vi "Main.vi"() -> ()   [LabVIEW 2017]
uses:
  Variable globale.vi
  ICNC/ICNC2.lvlib
panel:
  out "Speed Z":dbl
  out "Speed X":dbl
  out "Speed Y":dbl
  in  "Load Settings":bool
  in  "x-":bool
  in  "x+":bool
  out "Z Position":i32
  out "X Position":i32
  out "Y Position":i32
  in  "z+":bool
  in  "z-":bool
  in  "y+":bool
  in  "y-":bool
  in  "z+y+":bool
  in  "z-y+":bool
  in  "z-y-":bool
  in  "z+y-":bool
  in  "Speed in mm/s":dbl(slide) scale=0.0..1000.0
  in  "Go1":bool
  in  "Z":dbl
  in  "Y":dbl
  in  "X":dbl
  in  "System settings":bool
  out "Unlocked":bool
  out "Connected":bool
  in  "PARAM DLG":bool
  in  "stop motors":bool
  in  "Pos0":bool
  in  "stop":bool
  # "POSITION"
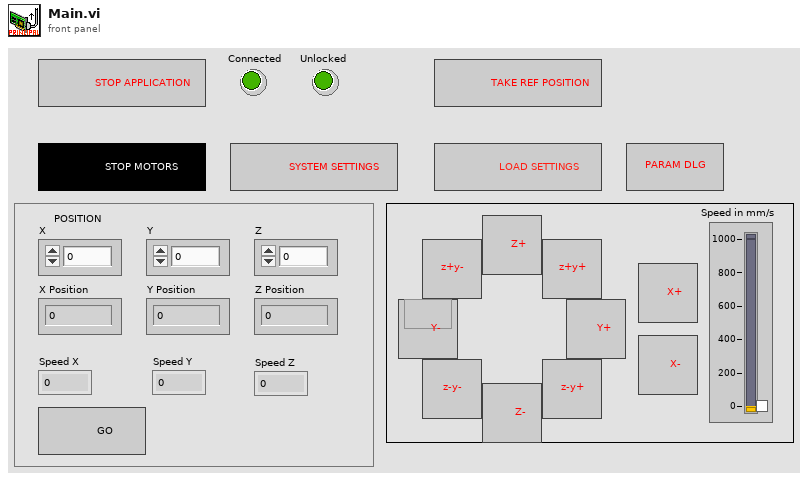
[diagram p1: front panel]
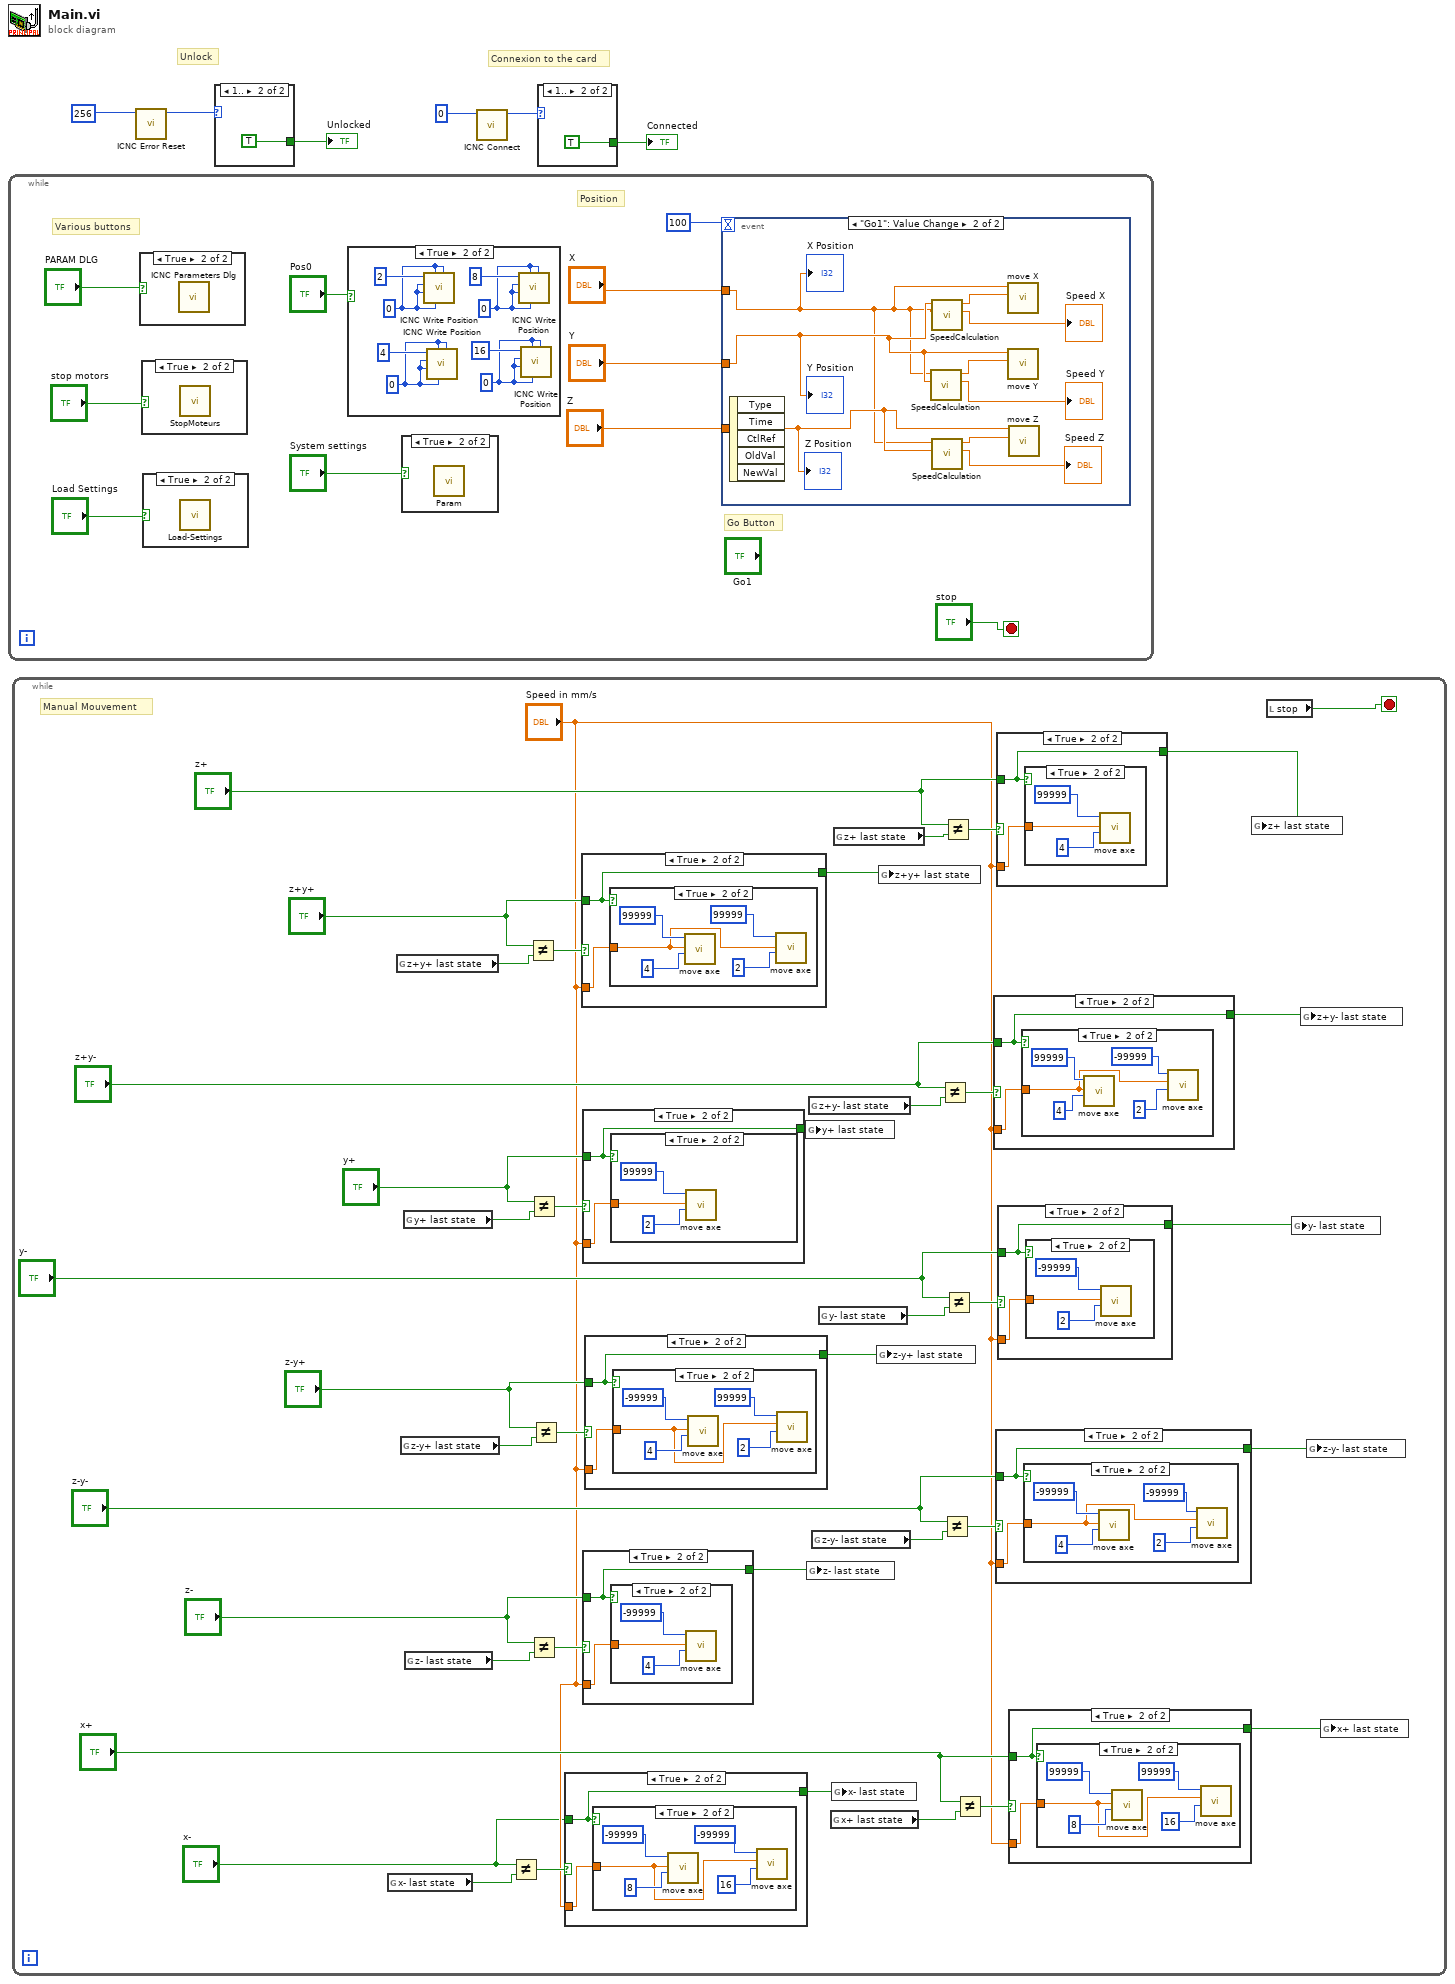
[diagram p0: block diagram]
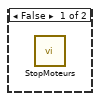
[diagram p3: hidden frame]
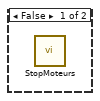
[diagram p5: hidden frame]
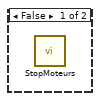
[diagram p7: hidden frame]
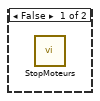
[diagram p9: hidden frame]
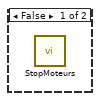
[diagram p11: hidden frame]
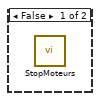
[diagram p13: hidden frame]
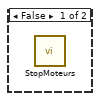
[diagram p15: hidden frame]
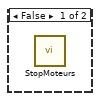
[diagram p17: hidden frame]
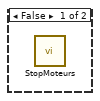
[diagram p19: hidden frame]
diagram:
  # "Connexion to the card"
  # "Unlock"
  n1 = while {
    stop <- "stop" stop-if-true
    # "Go Button"
    # "Various buttons"
    # "Position"
    n2 = case shown="True" "PARAM DLG" {
      frame False {
      }
      frame True {
        n3 = call "ICNC Parameters Dlg.vi"() -> ()  [unwired: 9 in, 3 out]
      }
    }
    n4 = case shown="True" "stop motors" {
      frame False {
      }
      frame True {
        n5 = call "StopMoteurs.vi"() -> ()  [unwired: 12 in]
      }
    }
    n6 = case shown="True" "Load Settings" {
      frame False {
      }
      frame True {
        n7 = call "Load-Settings.vi"() -> ()  [unwired: 12 in]
      }
    }
    n8 = case shown="True" "Pos0" {
      frame False {
      }
      frame True {
        w17 = 0
        w19 = 0
        w21 = 0
        w23 = 0
        n9 = call "ICNC Write Position.vi"("PositionB"=w23, "PositionA"=w23, "PositionZ"=w23, "PositionY"=w23, "PositionX"=w23, "Axis"=2) -> ()  [unwired: 4 in, 2 out]
        n10 = call "ICNC Write Position.vi"("PositionB"=w21, "PositionA"=w21, "PositionZ"=w21, "PositionY"=w21, "PositionX"=w21, "Axis"=4) -> ()  [unwired: 4 in, 2 out]
        n11 = call "ICNC Write Position.vi"("PositionB"=w19, "PositionA"=w19, "PositionZ"=w19, "PositionY"=w19, "PositionX"=w19, "Axis"=8) -> ()  [unwired: 4 in, 2 out]
        n12 = call "ICNC Write Position.vi"("PositionB"=w17, "PositionA"=w17, "PositionZ"=w17, "PositionY"=w17, "PositionX"=w17, "Axis"=16) -> ()  [unwired: 4 in, 2 out]
      }
    }
    n13 = case shown="True" "System settings" {
      frame False {
      }
      frame True {
        n14 = call "Param.vi"() -> ()  [unwired: 12 in]
      }
    }
    n15 = event shown="[1] \"Go1\": Value Change" {
      selector: _ -> [_ _]
      dyn-events: _ -> [_ _]
      timeout: 100 -> [_ _]
      tunnel: "X" -> [_ w27]
      tunnel: "Y" -> [_ w33]
      tunnel: "Z" -> [_ w28]
      event Timeout {
        n16 = event-data() -> ()  [unwired: 1 in, 2 out]
      }
      event "Go1": Value Change {
        n17 = event-data() -> ()  [unwired: 1 in, 5 out]
        n18 = call "SpeedCalculation.vi"("Axis1"=w33, "Axis2"=w27) -> ("Speed mm/s"=→"Speed Y":dbl, "Speed for card"=w32:dbl)  [unwired: 8 in]
        n19 = call "SpeedCalculation.vi"("Axis1"=w27, "Axis2"=w33) -> ("Speed mm/s"=→"Speed X":dbl, "Speed for card"=w31:dbl)  [unwired: 8 in]
        n20 = call "SpeedCalculation.vi"("Axis1"=w28, "Axis2"=w27) -> ("Speed mm/s"=→"Speed Z":dbl, "Speed for card"=w26:dbl)  [unwired: 8 in]
        n21 = call "move X.vi"("Speed X"=w31, "x mm"=w27) -> ()  [unwired: 10 in]
        n22 = call "move Y.vi"("Y Speed"=w32, "y mm"=w33) -> ()  [unwired: 10 in]
        n23 = call "move Z.vi"("Y Speed"=w26, "z mm"=w28) -> ()  [unwired: 10 in]
        "Y Position" <- w33
        "X Position" <- w27
        "Z Position" <- w28
      }
    }
  }
  n24 = while {
    stop <- w43 stop-if-true
    # "Manual Mouvement"
    n25 = global read "Variable globale.vi" "x- last state"() -> (w37:bool)
    n26 = global read "Variable globale.vi" "z+y+ last state"() -> (w70:bool)
    n27 = global read "Variable globale.vi" "z-y+ last state"() -> (w54:bool)
    n28 = global read "Variable globale.vi" "y+ last state"() -> (w62:bool)
    n29 = global read "Variable globale.vi" "z- last state"() -> (w66:bool)
    n30 = Not Equal?(x="x-", y=w37) -> (x != y?=w38:bool)
    n31 = Not Equal?(x="z+y+", y=w70) -> (x != y?=w71:bool)
    n32 = Not Equal?(x="y+", y=w62) -> (x != y?=w63:bool)
    n33 = Not Equal?(x="z-", y=w66) -> (x != y?=w67:bool)
    n34 = Not Equal?(x="z-y+", y=w54) -> (x != y?=w55:bool)
    n35 = case shown="True" w38 {
      tunnel: "Speed in mm/s" -> [_ w78]
      tunnel: "x-" -> [w76 w77]
      tunnel: [w76 w77] -> w36
      frame False {
      }
      frame True {
        n36 = case shown="True" w77 {
          tunnel: w78 -> [_ w79]
          frame False {
            n37 = call "StopMoteurs.vi"() -> ()  [unwired: 12 in]
          }
          frame True {
            n38 = call "move axe.vi"("Axe"=8, "Speed"=w79, "Angle"=-99999) -> ()  [unwired: 9 in]
            n39 = call "move axe.vi"("Axe"=16, "Speed"=w79, "Angle"=-99999) -> ()  [unwired: 9 in]
          }
        }
      }
    }
    n40 = case shown="True" w71 {
      tunnel: "Speed in mm/s" -> [_ w136]
      tunnel: "z+y+" -> [w134 w135]
      tunnel: [w134 w135] -> w69
      frame False {
      }
      frame True {
        n41 = case shown="True" w135 {
          tunnel: w136 -> [_ w138]
          frame False {
            n42 = call "StopMoteurs.vi"() -> ()  [unwired: 12 in]
          }
          frame True {
            n43 = call "move axe.vi"("Axe"=4, "Speed"=w138, "Angle"=99999) -> ()  [unwired: 9 in]
            n44 = call "move axe.vi"("Axe"=2, "Speed"=w138, "Angle"=99999) -> ()  [unwired: 9 in]
          }
        }
      }
    }
    n45 = case shown="True" w63 {
      tunnel: "Speed in mm/s" -> [_ w124]
      tunnel: "y+" -> [w122 w123]
      tunnel: [w122 w123] -> w61
      frame False {
      }
      frame True {
        n46 = case shown="True" w123 {
          tunnel: w124 -> [_ w126]
          frame False {
            n47 = call "StopMoteurs.vi"() -> ()  [unwired: 12 in]
          }
          frame True {
            n48 = call "move axe.vi"("Axe"=2, "Speed"=w126, "Angle"=99999) -> ()  [unwired: 9 in]
          }
        }
      }
    }
    n49 = case shown="True" w67 {
      tunnel: "Speed in mm/s" -> [_ w130]
      tunnel: "z-" -> [w128 w129]
      tunnel: [w128 w129] -> w65
      frame False {
      }
      frame True {
        n50 = case shown="True" w129 {
          tunnel: w130 -> [_ w132]
          frame False {
            n51 = call "StopMoteurs.vi"() -> ()  [unwired: 12 in]
          }
          frame True {
            n52 = call "move axe.vi"("Axe"=4, "Speed"=w132, "Angle"=-99999) -> ()  [unwired: 9 in]
          }
        }
      }
    }
    n53 = case shown="True" w55 {
      tunnel: "Speed in mm/s" -> [_ w108]
      tunnel: "z-y+" -> [w106 w107]
      tunnel: [w106 w107] -> w53
      frame False {
      }
      frame True {
        n54 = case shown="True" w107 {
          tunnel: w108 -> [_ w109]
          frame False {
            n55 = call "StopMoteurs.vi"() -> ()  [unwired: 12 in]
          }
          frame True {
            n56 = call "move axe.vi"("Axe"=4, "Speed"=w109, "Angle"=-99999) -> ()  [unwired: 9 in]
            n57 = call "move axe.vi"("Axe"=2, "Speed"=w109, "Angle"=99999) -> ()  [unwired: 9 in]
          }
        }
      }
    }
    n58 = global write "Variable globale.vi" "y+ last state"(w61) -> ()
    n59 = global write "Variable globale.vi" "z- last state"(w65) -> ()
    n60 = global read "Variable globale.vi" "z+y- last state"() -> (w58:bool)
    n61 = global read "Variable globale.vi" "z-y- last state"() -> (w46:bool)
    n62 = global read "Variable globale.vi" "y- last state"() -> (w50:bool)
    n63 = global read "Variable globale.vi" "x+ last state"() -> (w41:bool)
    n64 = global write "Variable globale.vi" "x- last state"(w36) -> ()
    n65 = global read "Variable globale.vi" "z+ last state"() -> (w74:bool)
    n66 = global write "Variable globale.vi" "z-y+ last state"(w53) -> ()
    n67 = global write "Variable globale.vi" "z+y+ last state"(w69) -> ()
    n68 = Not Equal?(x="z+y-", y=w58) -> (x != y?=w59:bool)
    n69 = Not Equal?(x="z-y-", y=w46) -> (x != y?=w47:bool)
    n70 = Not Equal?(x="z+", y=w74) -> (x != y?=w75:bool)
    n71 = Not Equal?(x="y-", y=w50) -> (x != y?=w51:bool)
    n72 = Not Equal?(x="x+", y=w41) -> (x != y?=w42:bool)
    n73 = case shown="True" w59 {
      tunnel: "Speed in mm/s" -> [_ w116]
      tunnel: "z+y-" -> [w114 w115]
      tunnel: [w114 w115] -> w57
      frame False {
      }
      frame True {
        n74 = case shown="True" w115 {
          tunnel: w116 -> [_ w117]
          frame False {
            n75 = call "StopMoteurs.vi"() -> ()  [unwired: 12 in]
          }
          frame True {
            n76 = call "move axe.vi"("Axe"=4, "Speed"=w117, "Angle"=99999) -> ()  [unwired: 9 in]
            n77 = call "move axe.vi"("Axe"=2, "Speed"=w117, "Angle"=-99999) -> ()  [unwired: 9 in]
          }
        }
      }
    }
    n78 = case shown="True" w47 {
      tunnel: "Speed in mm/s" -> [_ w94]
      tunnel: "z-y-" -> [w92 w93]
      tunnel: [w92 w93] -> w45
      frame False {
      }
      frame True {
        n79 = case shown="True" w93 {
          tunnel: w94 -> [_ w95]
          frame False {
            n80 = call "StopMoteurs.vi"() -> ()  [unwired: 12 in]
          }
          frame True {
            n81 = call "move axe.vi"("Axe"=4, "Speed"=w95, "Angle"=-99999) -> ()  [unwired: 9 in]
            n82 = call "move axe.vi"("Axe"=2, "Speed"=w95, "Angle"=-99999) -> ()  [unwired: 9 in]
          }
        }
      }
    }
    n83 = case shown="True" w75 {
      tunnel: "Speed in mm/s" -> [_ w144]
      tunnel: "z+" -> [w142 w143]
      tunnel: [w142 w143] -> w73
      frame False {
      }
      frame True {
        n84 = case shown="True" w143 {
          tunnel: w144 -> [_ w146]
          frame False {
            n85 = call "StopMoteurs.vi"() -> ()  [unwired: 12 in]
          }
          frame True {
            n86 = call "move axe.vi"("Axe"=4, "Speed"=w146, "Angle"=99999) -> ()  [unwired: 9 in]
          }
        }
      }
    }
    n87 = case shown="True" w51 {
      tunnel: "Speed in mm/s" -> [_ w102]
      tunnel: "y-" -> [w100 w101]
      tunnel: [w100 w101] -> w49
      frame False {
      }
      frame True {
        n88 = case shown="True" w101 {
          tunnel: w102 -> [_ w104]
          frame False {
            n89 = call "StopMoteurs.vi"() -> ()  [unwired: 12 in]
          }
          frame True {
            n90 = call "move axe.vi"("Axe"=2, "Speed"=w104, "Angle"=-99999) -> ()  [unwired: 9 in]
          }
        }
      }
    }
    n91 = case shown="True" w42 {
      tunnel: "Speed in mm/s" -> [_ w86]
      tunnel: "x+" -> [w84 w85]
      tunnel: [w84 w85] -> w40
      frame False {
      }
      frame True {
        n92 = case shown="True" w85 {
          tunnel: w86 -> [_ w87]
          frame False {
            n93 = call "StopMoteurs.vi"() -> ()  [unwired: 12 in]
          }
          frame True {
            n94 = call "move axe.vi"("Axe"=8, "Speed"=w87, "Angle"=99999) -> ()  [unwired: 9 in]
            n95 = call "move axe.vi"("Axe"=16, "Speed"=w87, "Angle"=99999) -> ()  [unwired: 9 in]
          }
        }
      }
    }
    n96 = global write "Variable globale.vi" "z+ last state"(w73) -> ()
    n97 = local read "stop"() -> (w43:bool)
    n98 = global write "Variable globale.vi" "y- last state"(w49) -> ()
    n99 = global write "Variable globale.vi" "z+y- last state"(w57) -> ()
    n100 = global write "Variable globale.vi" "z-y- last state"(w45) -> ()
    n101 = global write "Variable globale.vi" "x+ last state"(w40) -> ()
  }
  n102 = call "ICNC Error Reset.vi"("ErrorBits"=256) -> ("function return"=w2:u32)  [unwired: 9 in, 1 out]
  n103 = case shown="1.." w2 {
    tunnel: [FALSE TRUE] -> w5
    frame ..0 {
    }
    frame 1.. {
    }
  }
  "Unlocked" <- w5
  n104 = call "ICNC Connect.vi"("ICNC_Number"=0) -> ("function return"=w3:u32)  [unwired: 9 in, 1 out]
  n105 = case shown="1.." w3 {
    tunnel: [FALSE TRUE] -> w6
    frame ..0 {
    }
    frame 1.. {
    }
  }
  "Connected" <- w6
